vi "oax_gsBuild Data Path.vi"(2 "last path":path, 3 "Select Data":i32(listbox)) -> (0 "file path":path, 1 "Selected File":string)   [LabVIEW 2017]
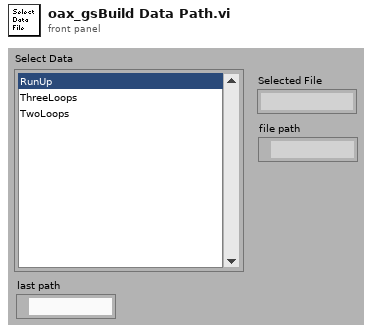
[diagram p1: front panel]
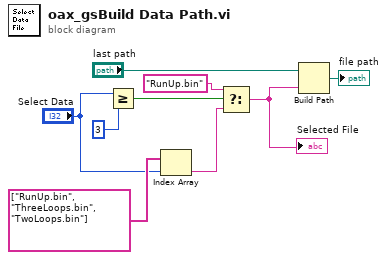
[diagram p0: block diagram]
diagram:
  n1 = Greater Or Equal?(x="Select Data", y=3) -> (x >= y?=w8:bool)
  n2 = Index Array(array=string[] ["RunUp.bin", "ThreeLoops.bin", "TwoLoops.bin"], index="Select Data") -> (element=w1:string)
  n3 = Select(t="RunUp.bin" ("f"), s=w8, f=w1) -> (s? t:f=w5:string)
  "Selected File" <- w5
  n4 = Build Path(base path="last path", name or relative path=w5) -> (appended path=→"file path":path)
